vi "Read configuration.vi"(8 "error in":errorcluster, 11 "MotionModule editor node in":refnum<class "MotionModule editor node.lvclass">) -> (0 "error out":errorcluster, 2 "configuration":refnum<class "NISE_CEF_serializable configuration.lvclass">, 3 "MotionModule editor node out":refnum<class "MotionModule editor node.lvclass">)   [LabVIEW 2017, in "MotionModule editor node.lvclass"]
uses:
  MotionModule editor node.lvclass
  <vilib>/NI/Configuration Framework/serializable configuration/NISE_CEF_serializable configuration.lvclass
  MotionModule editor node.lvclass/MotionModule editor node.ctl
  module/configuration/MotionModule configuration.lvclass
  C:/Program Files (x86)/National Instruments/LabVIEW 2017/vi.lib/NI/Configuration Framework/serializable configuration/NISE_CEF_serializable configuration.lvclass
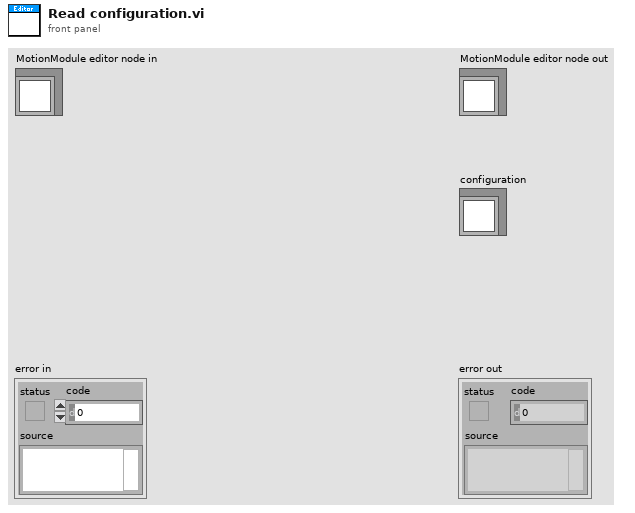
[diagram p1: front panel]
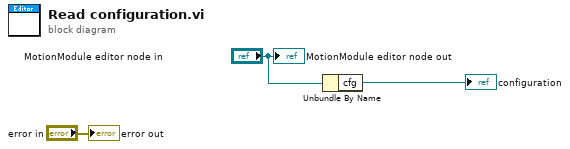
[diagram p0: block diagram]
diagram:
  n1 = Unbundle By Name("MotionModule editor node in") -> ("cfg"=→"configuration":refnum<class "MotionModule configuration.lvclass">)
  "error out" <- "error in"
  "MotionModule editor node out" <- "MotionModule editor node in"
